vi "Get Pending IMatch Responses.vi"(8 "error in":errorcluster, 11 "Response Matcher in":refnum<class "Node Guard.lvclass">) -> (0 "error out":errorcluster, 2 "Pending IMatch Responses":refnum<data-value>, 3 "Response Matcher out":refnum<class "Node Guard.lvclass">)   [LabVIEW 2024]
uses:
  Node Guard.lvclass/Node Guard.ctl
  Node Guard.lvclass
  C:/Program Files/National Instruments/LabVIEW 2026/vi.lib/ActorFramework/Actor/Actor.lvclass
  D:/git/CANopen-LabVIEW/source/Network Management/Node Guard/Node Guard.lvclass
  IResponse/IMatch Response.lvclass
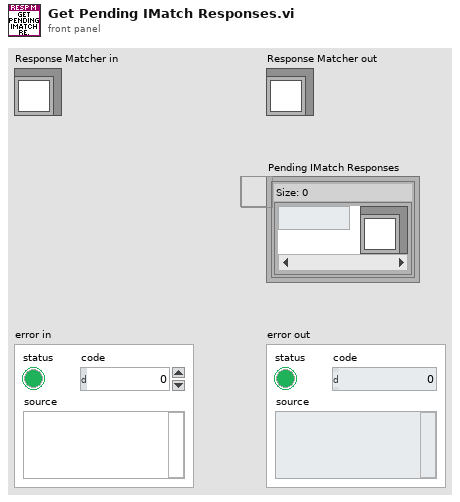
[diagram p1: front panel]
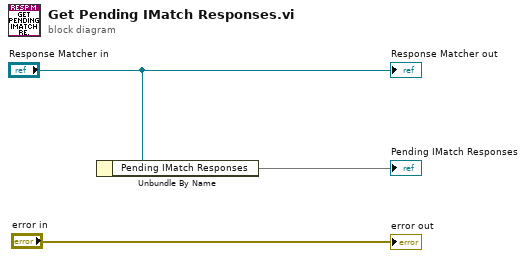
[diagram p0: block diagram]
diagram:
  n1 = Unbundle By Name("Response Matcher in") -> ("Pending IMatch Responses"=→"Pending IMatch Responses")
  "error out" <- "error in"
  "Response Matcher out" <- "Response Matcher in"
